vi "LWXPS_ControllerSlaveStatusStringGet.vi"(0 "XPS Reference IN":refnum<k24>, 7 "Slave Controller Status Code":i32, 11 "LabVIEW error IN":errorcluster) -> (4 "XPS Reference OUT":refnum<k24>, 6 "Returned error code":i32, 8 "Slave Controller Status String":string, 10 "XPS Error String":string, 15 "LabVIEW error OUT":errorcluster)   [LabVIEW 2014]
uses:
  D:/XPSQ8_LabView_Library/Development/Source/Dll/Newport.XPS.CommandInterface.dll
  Dll/Newport.XPS.CommandInterface.dll
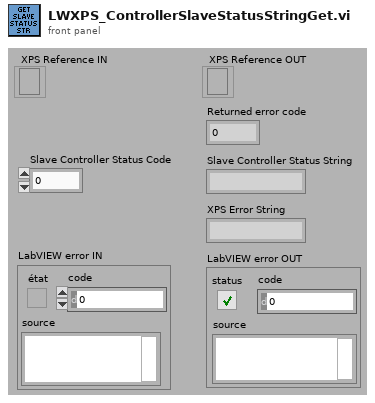
[diagram p1: front panel]
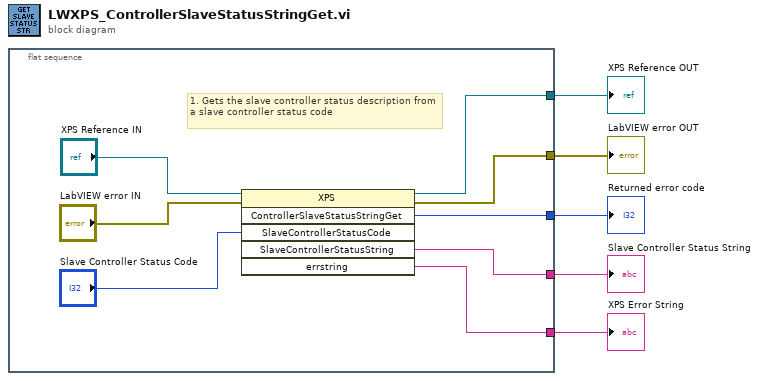
[diagram p0: block diagram]
diagram:
  n1 = flat-sequence {
    tunnel: [w10] -> w5
    tunnel: [w13] -> w4
    tunnel: [w11] -> w1
    tunnel: [w8] -> w2
    tunnel: [w9] -> w3
    frame #0 {
      # "1. Gets the slave controller status description from a slave controller status code"
      n2 = invoke class="XPS" method="ControllerSlaveStatusStringGet"(reference="XPS Reference IN", error in="LabVIEW error IN", "SlaveControllerStatusCode"="Slave Controller Status Code") -> (reference out=w10:refnum<k24>, error out=w13:errorcluster, "ControllerSlaveStatusStringGet"=w11:i32, "SlaveControllerStatusString"=w8:string, "errstring"=w9:string)  [unwired: 3 in, 1 out]
    }
  }
  "XPS Reference OUT" <- w5
  "LabVIEW error OUT" <- w4
  "XPS Error String" <- w3
  "Slave Controller Status String" <- w2
  "Returned error code" <- w1
